vi "SyncInit.vi"   [LabVIEW 2015]
uses:
  <instrlib>/niSync/niSync.llb/niSync Initialize (IVI).vi
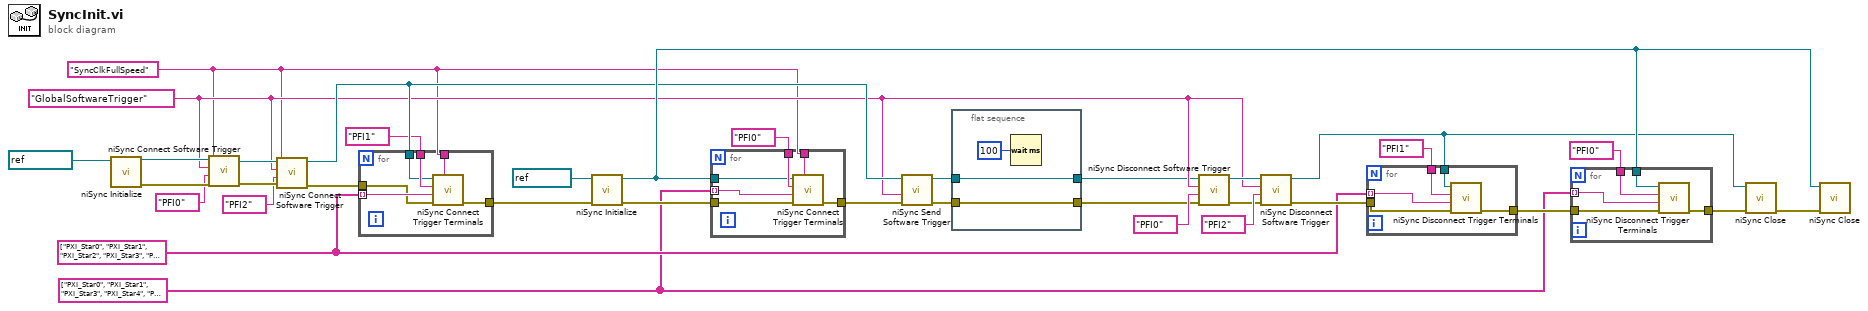
[diagram p0: block diagram]
diagram:
  w2 = string[] ["PXI_Star0", "PXI_Star1", "PXI_Star2", "PXI_Star3", "PXI_Star4"]
  w1 = string[] ["PXI_Star0", "PXI_Star1", "PXI_Star3", "PXI_Star4", "PXI_Star5", "PXI_Star6"]
  w7 = "SyncClkFullSpeed" ("synchronization clock")
  w8 = "GlobalSoftwareTrigger" ("source terminal")
  n1 = call-poly <instrlib>:"niSync Initialize.vi"("resource name"=refnum<k15> "Sync") -> ("error out"=w13:errorcluster, "instrument handle out"=w14:refnum<k15>)  [unwired: 2 in, 7 out]
  n2 = call <instrlib>:"niSync Connect Software Trigger.vi"("synchronization clock"=w7, "error in (no error)"=w13, "destination terminal"="PFI0", "source terminal"=w8, "instrument handle"=w14) -> ("error out"=w10:errorcluster, "instrument handle out"=w11:refnum<k15>)  [unwired: 2 in, 3 out]
  n3 = call <instrlib>:"niSync Connect Software Trigger.vi"("synchronization clock"=w7, "error in (no error)"=w10, "destination terminal"="PFI2", "source terminal"=w8, "instrument handle"=w11) -> ("error out"=w19:errorcluster, "instrument handle out"=w23:refnum<k15>)  [unwired: 2 in, 3 out]
  n4 = for {
    tunnel: "PFI1" ("source terminal") -> [w41]
    tunnel: w7 -> [w40]
    tunnel: w2 -> [w39] mode=indexing
    tunnel: w23 -> [w38]
    tunnel: w19 -> [w37]
    tunnel: [w36] -> w21
    n5 = call <instrlib>:"niSync Connect Trigger Terminals.vi"("synchronization clock"=w40, "error in (no error)"=w37, "destination terminal"=w39, "source terminal"=w41, "instrument handle"=w38) -> ("error out"=w36:errorcluster)  [unwired: 5 in, 1 out]
  }
  n6 = call-poly <instrlib>:"niSync Initialize.vi"("error in (no error)"=w21, "resource name"=refnum<k15> "Sync1") -> ("error out"=w20:errorcluster, "instrument handle out"=w35:refnum<k15>)  [unwired: 1 in, 7 out]
  n7 = for {
    tunnel: "PFI0" ("source terminal") -> [w47]
    tunnel: w7 -> [w46]
    tunnel: w1 -> [w45] mode=indexing
    tunnel: w35 -> [w44]
    tunnel: w20 -> [w43]
    tunnel: [w42] -> w22
    n8 = call <instrlib>:"niSync Connect Trigger Terminals.vi"("synchronization clock"=w46, "error in (no error)"=w43, "destination terminal"=w45, "source terminal"=w47, "instrument handle"=w44) -> ("error out"=w42:errorcluster)  [unwired: 5 in, 1 out]
  }
  n9 = call <instrlib>:"niSync Send Software Trigger.vi"("error in (no error)"=w22, "source terminal"=w8, "instrument handle"=w23) -> ("error out"=w6:errorcluster, "instrument handle out"=w3:refnum<k15>)  [unwired: 7 in]
  n10 = flat-sequence {
    tunnel: w6 -> [w50]
    tunnel: [w50] -> w5
    tunnel: [w49] -> w4
    tunnel: w3 -> [w49]
    frame #0 {
      n11 = Wait (ms)(milliseconds to wait=u32 100) -> ()  [unwired: 1 out]
    }
  }
  n12 = call <instrlib>:"niSync Disconnect Software Trigger.vi"("error in (no error)"=w5, "destination terminal"="PFI0", "source terminal"=w8, "instrument handle"=w4) -> ("error out"=w25:errorcluster, "instrument handle out"=w24:refnum<k15>)  [unwired: 6 in]
  n13 = call <instrlib>:"niSync Disconnect Software Trigger.vi"("error in (no error)"=w25, "destination terminal"="PFI2", "source terminal"=w8, "instrument handle"=w24) -> ("error out"=w29:errorcluster, "instrument handle out"=w34:refnum<k15>)  [unwired: 6 in]
  n14 = for {
    tunnel: "PFI1" ("source terminal") -> [w55]
    tunnel: w2 -> [w54] mode=indexing
    tunnel: w29 -> [w53]
    tunnel: w34 -> [w52]
    tunnel: [w51] -> w31
    n15 = call <instrlib>:"niSync Disconnect Trigger Terminals.vi"("error in (no error)"=w53, "destination terminal"=w54, "source terminal"=w55, "instrument handle"=w52) -> ("error out"=w51:errorcluster)  [unwired: 6 in, 1 out]
  }
  n16 = for {
    tunnel: "PFI0" ("source terminal") -> [w60]
    tunnel: w1 -> [w59] mode=indexing
    tunnel: w31 -> [w58]
    tunnel: [w57] -> w32
    tunnel: w35 -> [w56]
    n17 = call <instrlib>:"niSync Disconnect Trigger Terminals.vi"("error in (no error)"=w58, "destination terminal"=w59, "source terminal"=w60, "instrument handle"=w56) -> ("error out"=w57:errorcluster)  [unwired: 6 in, 1 out]
  }
  n18 = call <instrlib>:"niSync Close.vi"("error in (no error)"=w32, "instrument handle"=w34) -> ("error out"=w33:errorcluster)  [unwired: 9 in]
  n19 = call <instrlib>:"niSync Close.vi"("error in (no error)"=w33, "instrument handle"=w35) -> ()  [unwired: 9 in, 1 out]
